vi "serial_monitor_real2.vi"(1 "ON\nOFF":bool=TRUE caption="Init", 2 "Porta seriale":refnum<visa-resource-name>="COM3") -> ()   [LabVIEW 2014]
doc: "Lettura continua da porta seriale , INIT (true or false) della porta (9600, & bit, 1stop bit, EVEN)\nSalva su file\nFM&ADL aprile 2012"
uses:
  <vilib>/Instr/_visa.llb/VISA Configure Serial Port (Instr).vi
panel:
  in  "Baud rate":u32(ring)=9600 items=["9600"=9600, "14400"=14400, "19200"=19200, "38400"=38400, "57600"=57600, "115200"=115200]
  in  "SALVA I DATI SU FILE":bool=TRUE caption="ON\nOFF"
  out "Dati":dbl[][](graph)
  out "N_dati":u32
  out "lung":i32
  in  "stop":bool
  out "Number of Bytes at Serial Port":u32
  out "Dati trasmessi":string
  # "NO\nSI"
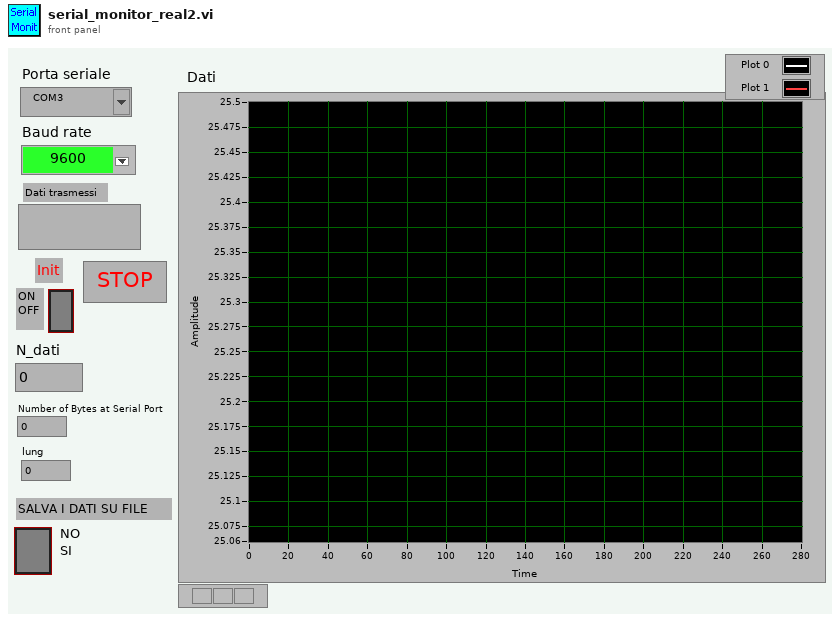
[diagram p1: front panel]
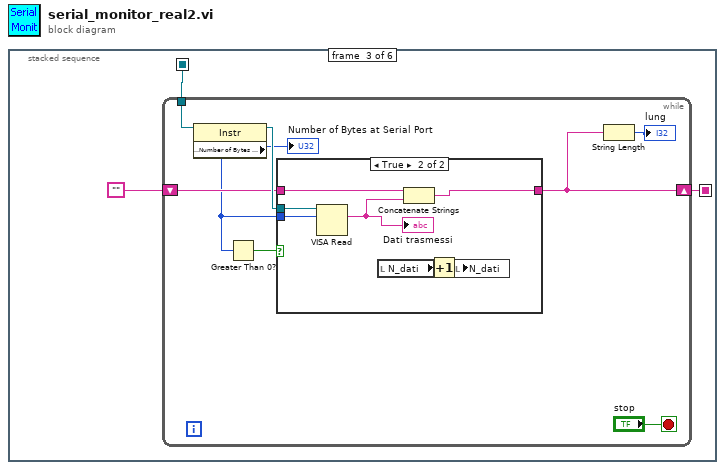
[diagram p0: block diagram]
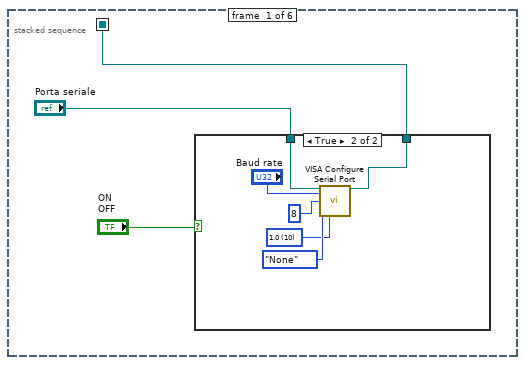
[diagram p2: hidden frame]
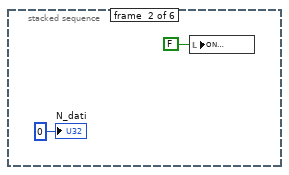
[diagram p4: hidden frame]
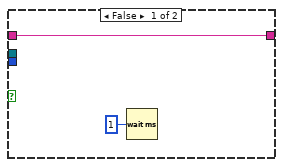
[diagram p5: hidden frame]
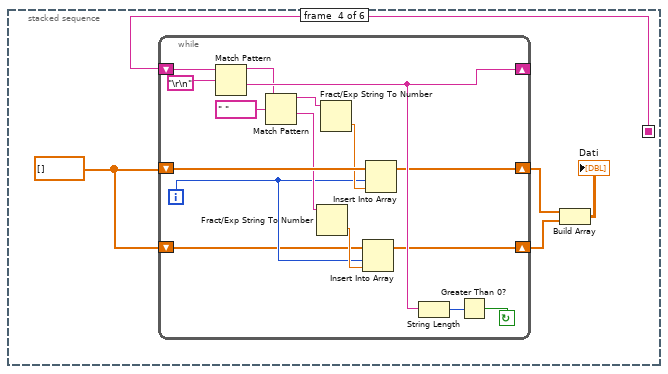
[diagram p6: hidden frame]
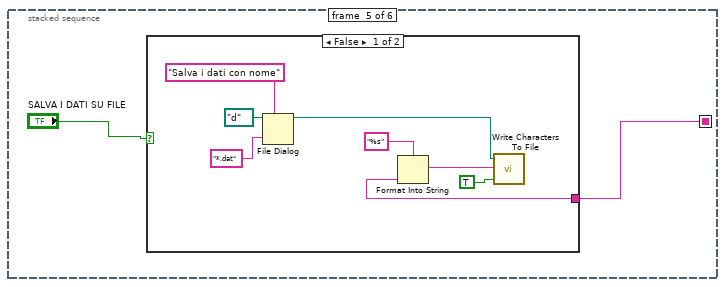
[diagram p7: hidden frame]
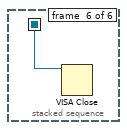
[diagram p9: hidden frame]
diagram:
  n1 = stacked-sequence {
    seq-local: [w1 _ _ _ _ _] -> [_ _ w15 _ _ w64]
    seq-local: [_ _ w13 _ _ _] -> [_ _ _ w37 w55 _]
    frame #0 {
      n2 = case shown="True" "ON\nOFF" {
        tunnel: "Porta seriale" -> [w4 w6]
        tunnel: [w4 w5] -> w1
        frame False {
        }
        frame True {
          w7 = u16 10 items=["1.0"=10, "1.5"=15, "2.0"=20] ("stop bits (10: 1 bit)")
          n3 = call-poly "VISA Configure Serial Port"("VISA resource name"=w6, "baud rate (9600)"="Baud rate", "data bits (8)"=u16 8, "parity (0:none)"=enum16{"None", "Odd", "Even", "Mark", "Space"}."None", "stop bits (10: 1 bit)"=w7) -> ("VISA resource name out"=w5:refnum<visa-resource-name>)  [unwired: 2 in, 8 out]
        }
      }
    }
    frame #1 {
      n4 = local write "ON\nOFF"(FALSE ("ON\nOFF")) -> ()
      "N_dati" <- u32 0 ("N_dati")
    }
    frame #2 {
      n5 = while {
        tunnel: w15 -> [w22]
        shift-right: [w16] -> w13
        shift-left: "" -> [w20]
        stop <- "stop" stop-if-true
        n6 = property class="Instr"(reference=w22) -> (reference out=w21:refnum<visa-resource-name>, "Serial Settings:Number of Bytes at Serial Port"=w17:u32)  [unwired: 1 in, 1 out]
        "Number of Bytes at Serial Port" <- w17
        n7 = Greater Than 0?(x=w17) -> (x > 0?=w18:bool)
        n8 = case shown="True" w18 {
          tunnel: w21 -> [_ w32]
          tunnel: w17 -> [_ w31]
          tunnel: w20 -> [w25 w30]
          tunnel: [w25 w29] -> w16
          frame False {
            n9 = Wait (ms)(milliseconds to wait=u32 1) -> ()  [unwired: 1 out]
          }
          frame True {
            n10 = VISA Read(VISA resource name=w32, byte count=w31) -> (read buffer=w28:string)  [unwired: 1 in, 3 out]
            "Dati trasmessi" <- w28
            n11 = local read "N_dati"() -> (w27:u32)
            n12 = Concatenate Strings(w30, w28) -> (w29:string)
            n13 = Increment(x=w27) -> (x+1=w26:u32)
            n14 = local write "N_dati"(w26) -> ()
          }
        }
        n15 = String Length(string=w16) -> (length=→"lung":i32)
      }
    }
    frame #3 {
      w36 = dbl[] []
      n16 = while {
        shift-right: [w47] -> w35
        shift-left: w36 -> [w48]
        shift-right: [w49] -> _
        shift-left: w37 -> [w50]
        shift-right: [w38] -> w34
        shift-left: w36 -> [w39]
        i -> [w40]
        stop <- w52 continue-if-true
        n17 = Match Pattern(string=w50, regular expression="\r\n") -> (before substring=w45:string, after substring=w49:string)  [unwired: 3 out]
        n18 = Match Pattern(string=w45, regular expression=" ") -> (before substring=w43:string, after substring=w42:string)  [unwired: 3 out]
        n19 = Fract/Exp String To Number(string=w42) -> (number=w41:dbl)  [unwired: 1 in, 3 out]
        n20 = Fract/Exp String To Number(string=w43) -> (number=w46:dbl)  [unwired: 1 in, 3 out]
        n21 = Insert Into Array(array=w39, index=w40, new element=w41) -> (w38:dbl[])
        n22 = Insert Into Array(array=w48, index=w40, new element=w46) -> (w47:dbl[])
        n23 = String Length(string=w49) -> (length=w53:i32)
        n24 = Greater Than 0?(x=w53) -> (x > 0?=w52:bool)
      }
      n25 = Build Array(w35, w34) -> (→"Dati":dbl[][])
    }
    frame #4 {
      n26 = case shown="False" "SALVA I DATI SU FILE" {
        tunnel: w55 -> [w63 _]
        frame False {
          n27 = File Dialog(6:"*.dat", 7:"Salva i dati con nome", 11:path "d:/" ("start path")) -> (3:w59:path)  [unwired: 1 in, 6 out]
          n28 = Format Into String(format string="%s", w63) -> (resulting string=w57:string)  [unwired: 2 in, 1 out]
          n29 = call <vilib>:"Write Characters To File.vi"("append to file? (new file:F)"=TRUE, "character string"=w57, "file path (dialog if empty)"=w59) -> ()  [unwired: 3 out]
        }
        frame True {
        }
      }
    }
    frame #5 {
      n30 = VISA Close(VISA resource name=w64) -> ()  [unwired: 1 in, 1 out]
    }
  }
